vi "A3200 Handler.vi"(8 "error in (no error)":errorcluster) -> (0 "error out":errorcluster, 3 "controller":refnum<k24>)   [LabVIEW 2026]
uses:
  <instrlib>/A3200/Bin/Aerotech.A3200.dll
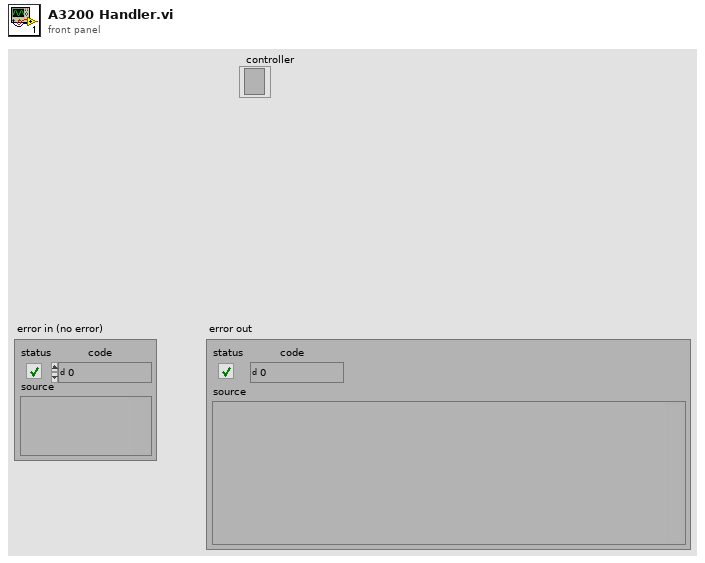
[diagram p1: front panel]
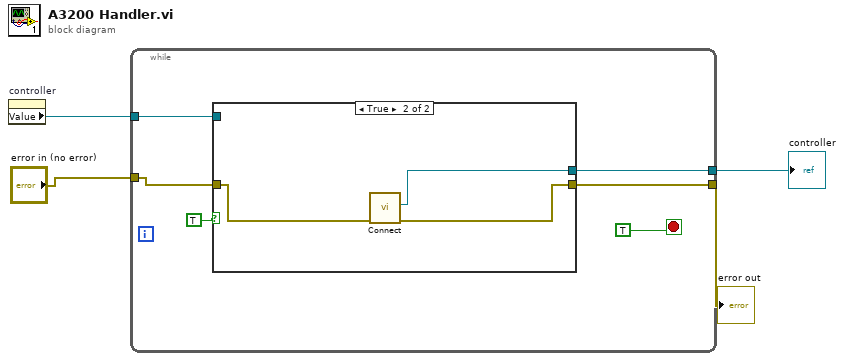
[diagram p0: block diagram]
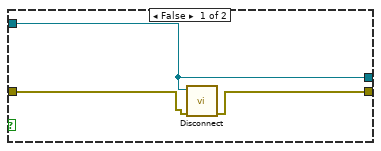
[diagram p2: hidden frame]
diagram:
  n1 = property on="controller" class="Ref (strict)"() -> ("Value"=w1:refnum<k24>)  [unwired: 2 in, 2 out]
  n2 = while {
    tunnel: "error in (no error)" -> [w10]
    tunnel: [w9] -> w3
    tunnel: [w8] -> w2
    tunnel: w1 -> [w7]
    stop <- TRUE stop-if-true
    n3 = case shown="True" TRUE {
      tunnel: w10 -> [w13 w16]
      tunnel: [w12 w15] -> w9
      tunnel: [w11 w14] -> w8
      tunnel: w7 -> [w11 _]
      frame False {
        n4 = call <instrlib>:"Disconnect.vi"("error in (no error)"=w13, "controller"=w11) -> ("error out"=w12:errorcluster)  [unwired: 9 in]
      }
      frame True {
        n5 = call <instrlib>:"Connect.vi"("error in (no error)"=w16) -> ("error out"=w15:errorcluster, "controller"=w14:refnum<k24>)  [unwired: 9 in]
      }
    }
  }
  "error out" <- w3
  "controller" <- w2
